vi "Create LLP Packet Timestamps.vi"(0 "serial input channel":string="SI0", 5 "llp packet sizes":u32[](array[numeric]), 7 "packet data types":T1[](array[typedef]), 9 "frame timing configuration":T2={"desired frame rate (fps)"=0.0, "actual link data rate (B/s)"=385000000.0, "minimum delay between packets (cycles)"=500, "line blanking (cycles)"=500} {"actual link data rate (B/s)" format="%_6p"; "line blanking (cycles)" format="%#_6p"}, 11 "error in (no error)":errorcluster, 12 "frame start timestamp":u64) -> (4 "timestamps":u64[](array[numeric]), 6 "actual frame rate (fps)":dbl, 8 "next frame start timestamp":u64, 15 "error out":errorcluster)   [LabVIEW 2023, in "GettingStarted_Gen_148X_Host.lvlib"]
uses:
  GettingStarted_Gen_148X_Host.lvlib
  Types/Frame Timing Configuration.ctl
  <instrlib>/FlexRIO/CSI-2/v2/Common/Types/LLP Data Type.ctl
  <instrlib>/FlexRIO/CSI-2/v2/FPGA/Types/FPGA LLP Packet Timestamp.ctl
  <instrlib>/FlexRIO/CSI-2/v2/FPGA/Types/Timestamp ID.ctl
  <instrlib>/FlexRIO/CSI-2/v2/FPGA/subVIs/Convert LLP Packet Timestamp to Raw Timestamp.vi
  <instrlib>/FlexRIO/CSI-2/v2/FPGA/NI CSI-2 API FPGA v2.lvlib
  FPGA/Common/GettingStarted_Common_148X_FPGA.lvlib
  <instrlib>/FlexRIO/Automotive Vision Utility/v1/Host/Automotive Vision Utility.lvlib
  <instrlib>/FlexRIO/CSI-2/v2/Common/NI CSI-2 API Common v2.lvlib
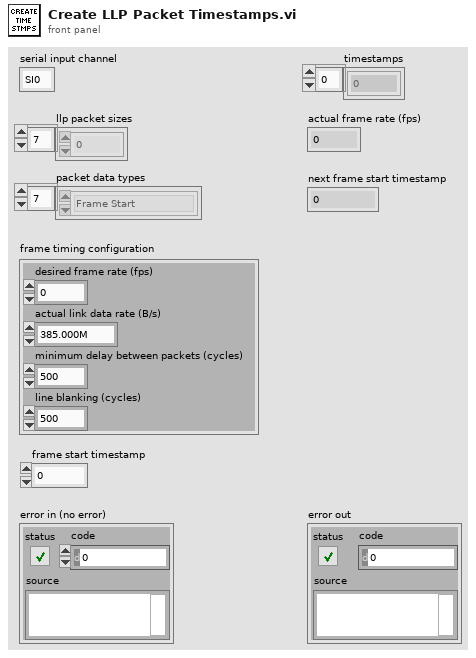
[diagram p1: front panel]
types:
  T1 = typedef "NI CSI-2 API Common v2.lvlib/LLP Data Type.ctl" = enum8{"Frame Start", "Frame End", "Line Start", "Line End", "End of Transmission", "Reserved 0", "Reserved 1", "Reserved 2", "Generic Short Packet 1", "Generic Short Packet 2", "Generic Short Packet 3", "Generic Short Packet 4", "Generic Short Packet 5", "Generic Short Packet 6", "Generic Short Packet 7", "Generic Short Packet 8", "Null", "Blanking Data", "Embedded 8-bit non Image Data", "Generic Long Packet 1", "Generic Long Packet 2", "Generic Long Packet 3", "Generic Long Packet 4", "Reserved 3", "YUV420 8-bit", "YUV420 10-bit", "Legacy YUV420 8-bit", "Reserved 4", "YUV420 8-bit Chroma Shifted", "YUV420 10-bit Chroma Shifted", "YUV422 8-bit", "YUV422 10-bit", "RGB444", "RGB555", "RGB565", "RGB666", "RGB888", "Reserved 5", "Reserved 6", "RAW 24", "RAW 6", "RAW 7", "RAW 8", "RAW 10", "RAW 12", "RAW 14", "RAW 16", "RAW 20", "User Defined 8-bit Data 1", "User Defined 8-bit Data 2", "User Defined 8-bit Data 3", "User Defined 8-bit Data 4", "User Defined 8-bit Data 5", "User Defined 8-bit Data 6", "User Defined 8-bit Data 7", "User Defined 8-bit Data 8", "USL Command", "Reserved 7", "Reserved 8", "Reserved 9", "Reserved 10", "Reserved 11", "Reserved 12", "LRTE EPD Spacer"}
  T2 = typedef "GettingStarted_Gen_148X_Host.lvlib/Frame Timing Configuration.ctl" = cluster{"desired frame rate (fps)":dbl, "actual link data rate (B/s)":dbl, "minimum delay between packets (cycles)":u64, "line blanking (cycles)":u64}
  T3 = typedef "Automotive Vision Utility.lvlib/Serial Channel Type.ctl" = enum16{"Serial Input Channel", "Serial Output Channel", "Unknown Channel Type"}
  T4 = typedef "NI CSI-2 API FPGA v2.lvlib/FPGA LLP Packet Timestamp.ctl" = cluster{"valid":bool, "count":fxp<+,50,50>, "id":T5, "metadata":u8}
  T5 = typedef "NI CSI-2 API FPGA v2.lvlib/Timestamp ID.ctl" = enum8{"SI0 LLP", "SI1 LLP", "SI2 LLP", "SI3 LLP", "SI4 LLP", "SI5 LLP", "SI6 LLP", "SI7 LLP", "SO0 LLP", "SO1 LLP", "SO2 LLP", "SO3 LLP", "SO4 LLP", "SO5 LLP", "SO6 LLP", "SO7 LLP", "Ser0 GPIO Bank", "Ser1 GPIO Bank", "Ser2 GPIO Bank", "Ser3 GPIO Bank", "Ser4 GPIO Bank", "Ser5 GPIO Bank", "Ser6 GPIO Bank", "Ser7 GPIO Bank", "Des0 GPIO Bank", "Des1 GPIO Bank", "Des2 GPIO Bank", "Des3 GPIO Bank", "Des4 GPIO Bank", "Des5 GPIO Bank", "Des6 GPIO Bank", "Des7 GPIO Bank", "User0", "User1", "User2", "User3", "User4", "User5", "User6", "User7", "User8", "User9", "User10", "User11", "User12", "User13", "User14", "User15", "User16", "User17", "User18", "User19", "User20", "User21", "User22", "User23", "User24", "User25", "User26", "User27", "User28", "User29", "User30", "User31"}
  T6 = typedef "NI CSI-2 API FPGA v2.lvlib/Raw Timestamp.ctl" = cluster{"timestamp":u64, "valid":bool}
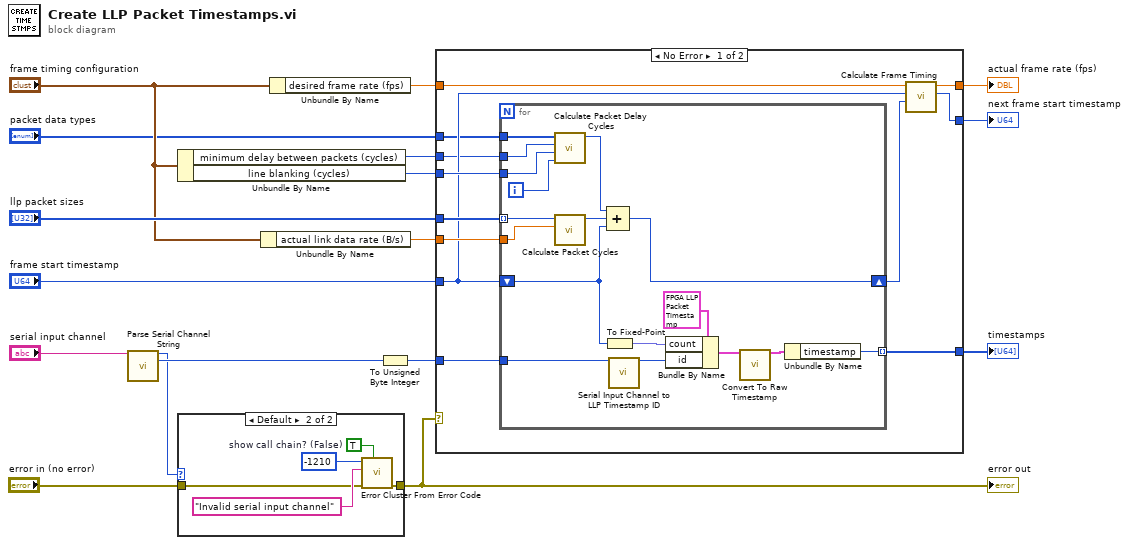
[diagram p0: block diagram]
diagram:
  n1 = call <instrlib>:"Parse Serial Channel String.vi"("serial channel string"="serial input channel") -> ("serial channel type"=w11:T3, "channel number"=w14:i32)  [unwired: 13 in]
  n2 = Unbundle By Name("frame timing configuration") -> ("minimum delay between packets (cycles)"=w2:u64, "line blanking (cycles)"=w7:u64)
  n3 = case shown="Default" w11 {
    tunnel: "error in (no error)" -> [w18 w20]
    tunnel: [w18 w19] -> w10
    frame "Serial Input Channel" {
    }
    frame Default {
      w21 = TRUE  # show call chain? (False)
      n4 = call <vilib>:"Error Cluster From Error Code.vi"("show call chain? (False)"=w21, "error in (no error)"=w20, "error message (\"\")"="Invalid serial input channel" ("error message (\"\")"), "error code (0)"=-1210) -> ("error out"=w19:errorcluster)  [unwired: 5 in]
    }
  }
  "error out" <- w10
  n5 = Unbundle By Name("frame timing configuration") -> ("actual link data rate (B/s)"=w8:dbl)
  n6 = Unbundle By Name("frame timing configuration") -> ("desired frame rate (fps)"=w6:dbl)
  n7 = To Unsigned Byte Integer(number=w14) -> (unsigned 8bit integer=w13:u8)
  n8 = case shown="No Error" w10 {
    tunnel: w7 -> [w35 _]
    tunnel: w8 -> [w34 _]
    tunnel: "llp packet sizes" -> [w33 _]
    tunnel: [w32 _] -> w16
    tunnel: w13 -> [w31 _]
    tunnel: "frame start timestamp" -> [w27 _]
    tunnel: w6 -> [w30 _]
    tunnel: [w28 _] -> w4
    tunnel: [w26 _] -> w3
    tunnel: w2 -> [w25 _]
    tunnel: "packet data types" -> [w24 _]
    frame No Error {
      n9 = for {
        tunnel: w33 -> [w43] mode=indexing
        tunnel: w34 -> [w52]
        shift-right: [w50] -> w29
        shift-left: w27 -> [w45]
        tunnel: w35 -> [w37]
        tunnel: [w44] -> w32 mode=indexing
        tunnel: w31 -> [w41]
        tunnel: w25 -> [w38]
        tunnel: w24 -> [w39]
        i -> [w36]
        n10 = call "Calculate Packet Delay Cycles.vi"("current packet  index"=w36, "line blanking (cycles)"=w37, "minimum delay between packets (cycles)"=w38, "packet data types"=w39) -> ("packet delay (cycles)"=w40:u64)  [unwired: 7 in]
        n11 = call "Calculate Packet Cycles.vi"("actual link data rate (B/s)"=w52, "packet size"=w43) -> ("packet cycles"=w51:u64)  [unwired: 9 in]
        n12 = To Fixed-Point(number=w45) -> (fixed-point=w42:fxp<+,50,50>)  [unwired: 1 in]
        n13 = Compound Arithmetic op=ADD(w40, w51, w45) -> (w50:u64)
        n14 = call "Serial Input Channel to LLP Timestamp ID.vi"("serial input channel instance"=w41) -> ("llp timestamp id"=w48:T5)  [unwired: 14 in]
        n15 = Bundle By Name(cluster=T4 {"valid"=FALSE, "count"=0.0, "id"=enum."SI0 LLP", "metadata"=0} ("LLP Packet Timestamp"), "count"=w42, "id"=w48) -> (w47:T4)
        n16 = call-poly <instrlib>:"Convert To Raw Timestamp.vi"("llp packet timestamp"=w47) -> ("raw timestamp"=w46:T6)  [unwired: 14 in]
        n17 = Unbundle By Name(w46) -> ("timestamp"=w44:u64)
      }
      n18 = call "Calculate Frame Timing.vi"("estimated next frame start timestamp"=w29, "frame start timestamp"=w27, "desired frame rate (fps)"=w30) -> ("actual next frame start timestamp"=w28:u64, "actual frame rate (fps)"=w26:dbl)  [unwired: 7 in]
    }
    frame Error {
    }
  }
  "timestamps" <- w16
  "next frame start timestamp" <- w4
  "actual frame rate (fps)" <- w3
